vi "PH_Sixpack_Switch.contents.vi"   [LabVIEW 2014, in "PH_Sixpack_Switch.lvlib"]
doc: "This class is forseen to control 6P applications used as a switch (driving between the \"outer\" (1) and \"inner\" (2) position. \n\nThis class is part of the PHELIX device layer."
uses:
  PH_Sixpack_Switch.lvlib
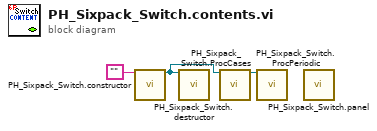
[diagram p0: block diagram]
diagram:
  n1 = call "PH_Sixpack_Switch.constructor.vi"("name"="") -> ("i ref out"=w1:refnum<vi>)  [unwired: 16 in, 2 out]
  n2 = call "PH_Sixpack_Switch.destructor.vi"("i ref in"=w1) -> ()  [unwired: 18 in, 1 out]
  n3 = call "PH_Sixpack_Switch.ProcCases.vi"("i ref in"=w1) -> ("i ref out"=w3:refnum<vi>)  [unwired: 16 in, 2 out]
  n4 = call "PH_Sixpack_Switch.ProcPeriodic.vi"("i ref in"=w3) -> ()  [unwired: 16 in, 3 out]
  n5 = call "PH_Sixpack_Switch.panel.vi"() -> ()  [unwired: 19 in, 1 out]
